vi "ConfigDevice.vi"(8 "error in (no error)":errorcluster, 11 "ChromaAcLoad in":refnum<class "ChromaAcLoad.lvclass">) -> (0 "error out":errorcluster, 3 "ChromaAcLoad out":refnum<class "ChromaAcLoad.lvclass">)   [LabVIEW 2018, in "AcPwrPlugins.lvlib" / "ChromaAcLoad.lvclass"]
doc: "This VI configures the instrument based on the INI file settings or changes to these settings made using the PrefDialog.vi."
uses:
  ChromaAcLoad.lvclass
  TypeDefs/RangeCheck.ctl
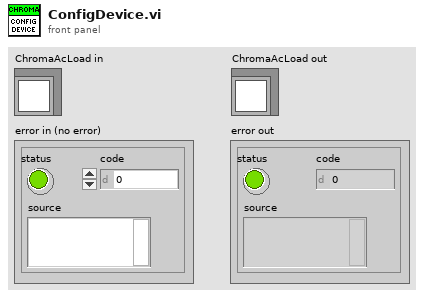
[diagram p1: front panel]
types:
  T1 = enum16{"Constant Voltage (DC)", "Constant Power (DC)", "Constant Power (AC)", "Constant Current (DC)", "Constant Current (AC)", "Constant Resistance (DC)", "Constant Resistance (AC)", "Rectified Mode (DC)", "Inrush (AC)", "RLC CP (AC)", "RLC (AC)"}
  T2 = cluster{"Handle":string, "Name":string, "Phase Select":i32, "Instrument Options":string, "id query (T)":bool, "reset device (T)":bool, "Load Short Circuited":bool, "Line Synchronization":bool, "Load Current (A/Arms)":dbl, "Load Voltage (V/Vrms)":dbl, "Load Power (W)":dbl, "Load Resistance (Ohms)":dbl, "Load Current Peak Limit (A)":dbl, "Load Current Limit (A/Arms)":dbl, "Load Power Limit (W)":dbl, "Synch Frequency (Hz)":dbl, "Priority":enum16{"CF Only", "PF Only", "Both (CF)", "Both (PF)"}, "Crest Factor":dbl, "Power Factor":dbl, "Slew Rate":cluster{"Rise Slew Rate (A/ms)":i32, "Fall Slew Rate (A/ms)":i32}, "LC/RLC Mode":cluster{"Capacitance (uF)":i32, "Inductance (uH)":i32, "Series Resistance (Ohm)":dbl, "Parallel Resistance (Ohm)":dbl}, "Timing":cluster{"TimingOn":enum16{""}, "Hours":u32, "Minutes":u32, "Seconds":dbl, "CutoffVoltage":dbl}, "Connected":bool}[]
  T3 = typedef "AcPwrPlugins.lvlib/ChromaAcLoad.lvclass/RangeCheck.ctl" = enum16{"Power", "Power Limit", "Current", "Current Peak", "Current Limit", "Voltage", "AC Resistance", "DC Resistance", "Frequency", "Crest Factor", "Power Factor", "RLC Power Factor", "Rise Slew Rate", "Fall Slew Rate", "Capacitance", "Inductance", "Parallel Resistance", "Series Resistance"}[]
  T4 = enum16{"CF Only", "PF Only", "Both (CF)", "Both (PF)"}
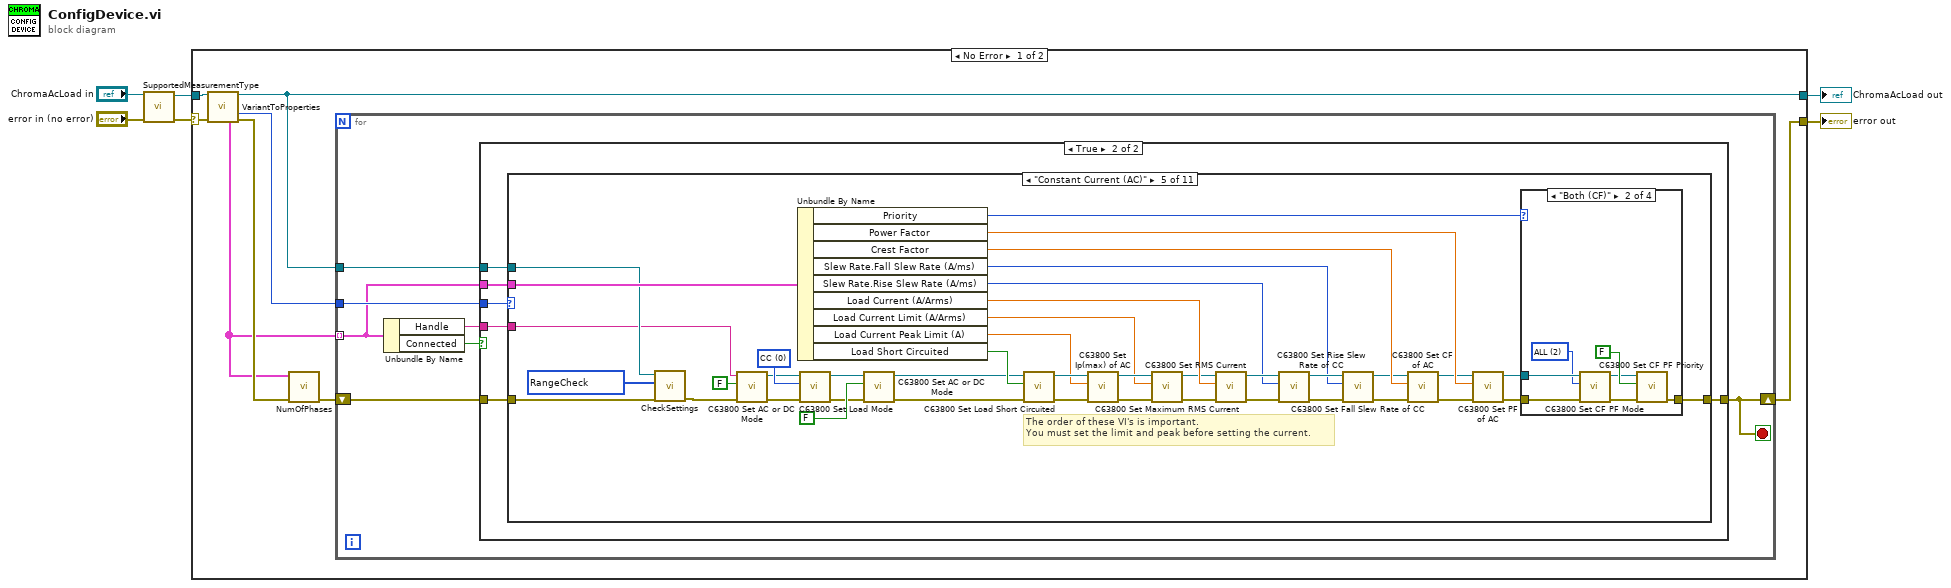
[diagram p0: block diagram]
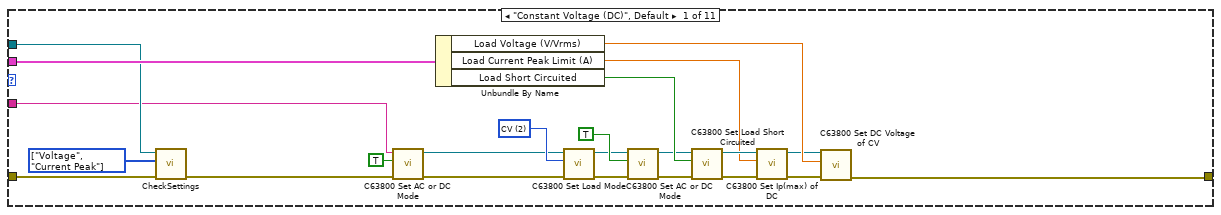
[diagram p3: hidden frame]
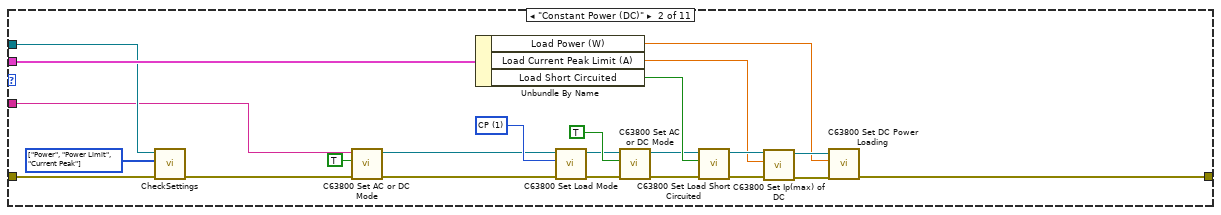
[diagram p4: hidden frame]
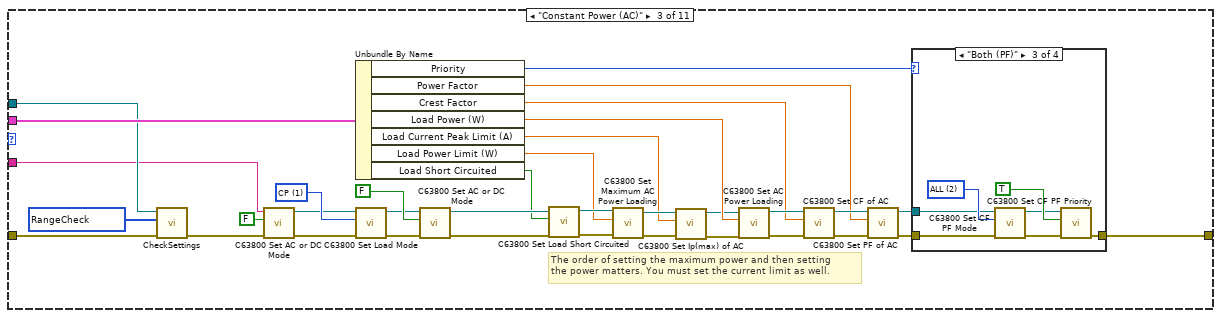
[diagram p5: hidden frame]
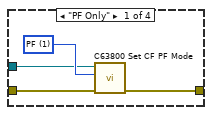
[diagram p6: hidden frame]
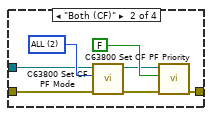
[diagram p7: hidden frame]
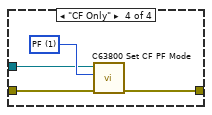
[diagram p8: hidden frame]
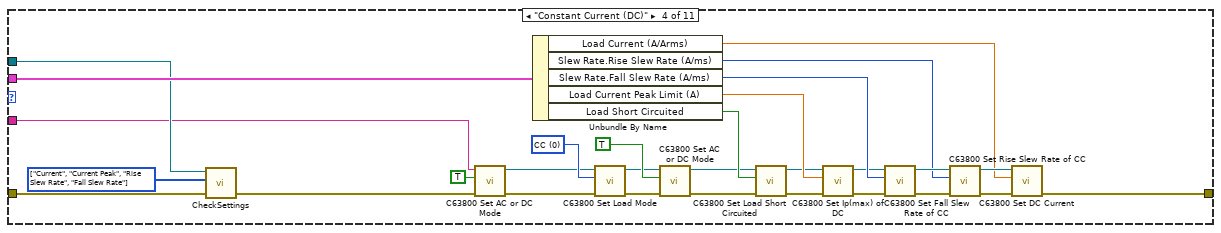
[diagram p9: hidden frame]
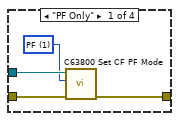
[diagram p10: hidden frame]
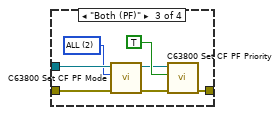
[diagram p11: hidden frame]
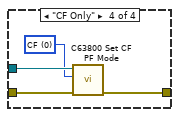
[diagram p12: hidden frame]
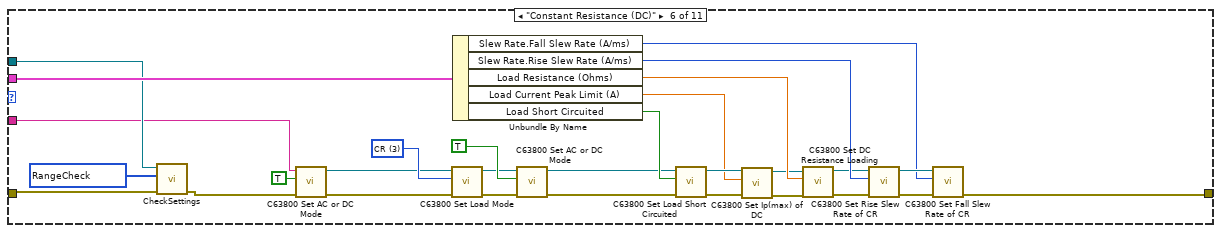
[diagram p13: hidden frame]
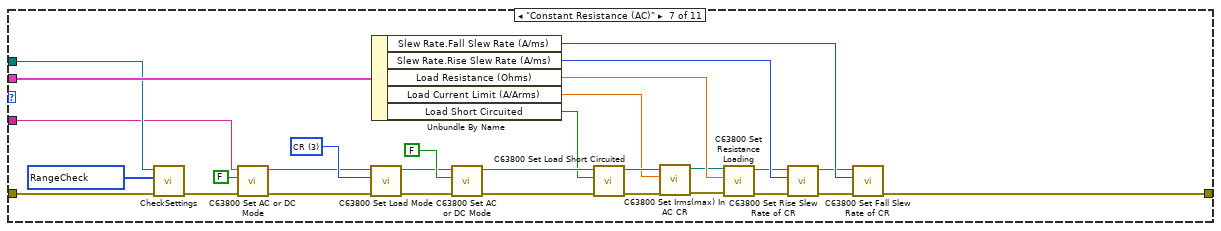
[diagram p14: hidden frame]
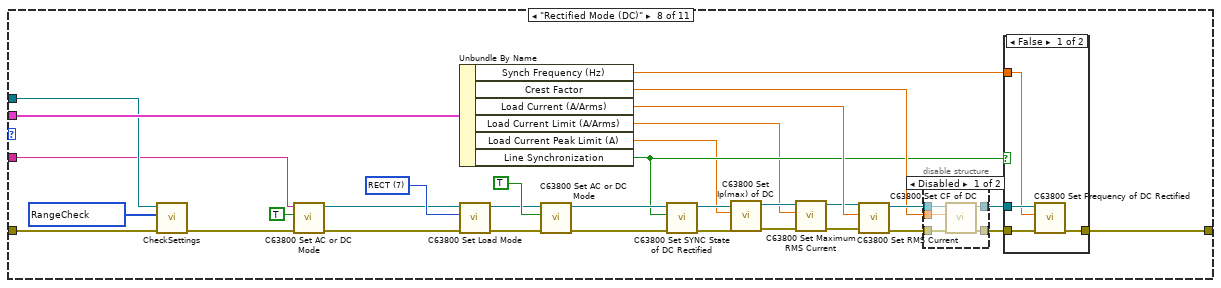
[diagram p15: hidden frame]
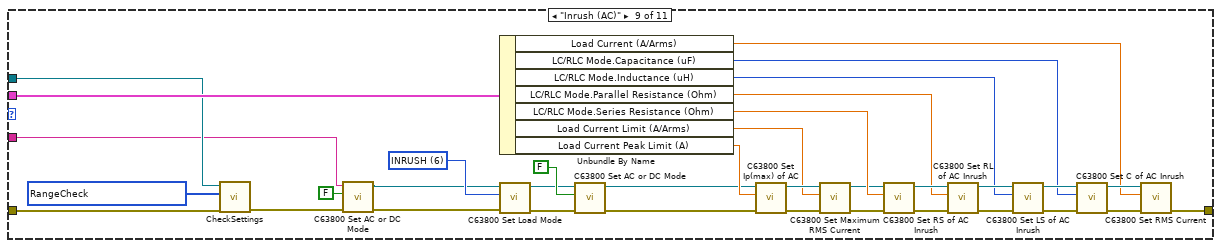
[diagram p18: hidden frame]
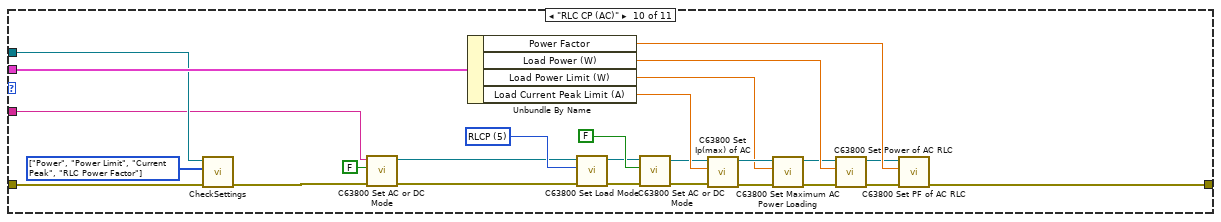
[diagram p19: hidden frame]
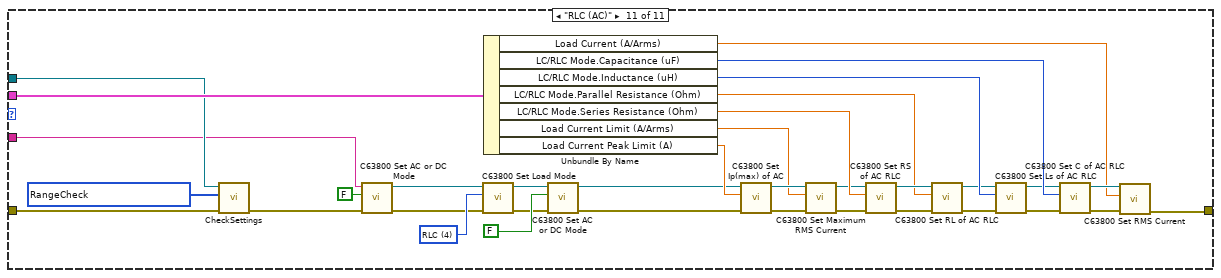
[diagram p20: hidden frame]
diagram:
  n1 = call-dynamic "SupportedMeasurementType.vi"("error in (no error)"="error in (no error)", "ChromaAcLoad in"="ChromaAcLoad in") -> ("error out"=w3:errorcluster, "ChromaAcLoad out"=w4:refnum<class "ChromaAcLoad.lvclass">)  [unwired: 8 in]
  n2 = case shown="No Error" w3 {
    selector: w3 -> [w11 w419]
    tunnel: [w14 w419] -> w6
    tunnel: w4 -> [w13 w418]
    tunnel: [w9 w418] -> w5
    frame No Error {
      n3 = call "VariantToProperties.vi"("ChromaAcLoad"=w13, "error in (no error)"=w11) -> ("ChromaAcLoad"=w9:refnum<class "ChromaAcLoad.lvclass">, "Configuration Mode"=w7:T1, "Phases"=w8:T2, "error out"=w10:errorcluster)  [unwired: 7 in, 3 out]
      n4 = call "NumOfPhases.vi"("Error In"=w10, "Phases"=w8) -> ("Error Out"=w12:errorcluster)  [unwired: 8 in, 1 out]
      n5 = for {
        shift-right: [w18] -> w14
        shift-left: w12 -> [w19]
        tunnel: w8 -> [w16] mode=indexing
        tunnel: w7 -> [w21]
        tunnel: w9 -> [w15]
        stop <- w18 stop-if-true
        n6 = Unbundle By Name(w16) -> ("Handle"=w17:string, "Connected"=w20:bool)
        n7 = case shown="True" w20 {
          tunnel: w21 -> [_ w26]
          tunnel: w19 -> [w22 w28]
          tunnel: [w22 w27] -> w18
          tunnel: w17 -> [_ w25]
          tunnel: w16 -> [_ w24]
          tunnel: w15 -> [_ w23]
          frame False {
          }
          frame True {
            n8 = case shown="\"Constant Current (AC)\"" w26 {
              tunnel: w28 -> [w41 w72 w107 w146 w179 w232 w269 w298 w337 w373 w400]
              tunnel: [w43 w71 w109 w137 w188 w241 w277 w305 w334 w369 w394] -> w27
              tunnel: w25 -> [w31 w54 w75 w130 w159 w221 w250 w278 w325 w357 w383]
              tunnel: w24 -> [w50 w74 w108 w153 w189 w239 w276 w304 w345 w381 w406]
              tunnel: w23 -> [w40 w73 w106 w145 w178 w231 w268 w297 w338 w372 w398]
              frame "Constant Voltage (DC)", Default {
                w39 = T3 [enum."Voltage", enum."Current Peak"] items=["Power", "Power Limit", "Current", "Current Peak", "Current Limit", "Voltage", "AC Resistance", "DC Resistance", "Frequency", "Crest Factor", "Power Factor", "RLC Power Factor", "Rise Slew Rate", "Fall Slew Rate", "Capacitance", "Inductance", "Parallel Resistance", "Series Resistance"] ("RangeCheck")
                w46 = 2 items=["CC", "CP", "CV", "CR", "RLC", "RLCP", "INRUSH", "RECT"] ("Load Mode")
                n9 = call-dynamic "CheckSettings.vi"("ChromaAcLoad in"=w40, "RangeCheck"=w39, "error in (no error)"=w41) -> ("error out"=w33:errorcluster)  [unwired: 6 in, 1 out]
                n10 = call <instrlib>:"C63800 Set AC or DC Mode.vi"("error in (no error)"=w33, "Select AC_DC Mode"=TRUE, "Instrument Handle"=w31) -> ("error out"=w32:errorcluster, "Instrument Handle out"=w30:refnum<k15>)  [unwired: 7 in]
                n11 = Unbundle By Name(w50) -> ("Load Voltage (V/Vrms)"=w42:dbl, "Load Current Peak Limit (A)"=w34:dbl, "Load Short Circuited"=w51:bool)
                n12 = call <instrlib>:"C63800 Set Load Mode.vi"("error in (no error)"=w32, "Load Mode"=w46, "Instrument Handle"=w30) -> ("error out"=w45:errorcluster, "Instrument Handle out"=w44:refnum<k15>)  [unwired: 7 in]
                n13 = call <instrlib>:"C63800 Set AC or DC Mode.vi"("error in (no error)"=w45, "Select AC_DC Mode"=TRUE, "Instrument Handle"=w44) -> ("error out"=w49:errorcluster, "Instrument Handle out"=w47:refnum<k15>)  [unwired: 7 in]
                n14 = call <instrlib>:"C63800 Set Load Short Circuited.vi"("error in (no error)"=w49, "Short Circuited State"=w51, "Instrument Handle"=w47) -> ("error out"=w38:errorcluster, "Instrument Handle out"=w35:refnum<k15>)  [unwired: 7 in]
                n15 = call <instrlib>:"C63800 Set Ip(max) of DC.vi"("error in (no error)"=w38, "I_max_DC"=w34, "Instrument Handle"=w35) -> ("error out"=w36:errorcluster, "Instrument Handle out"=w37:refnum<k15>)  [unwired: 7 in]
                n16 = call <instrlib>:"C63800 Set DC Voltage of CV.vi"("error in (no error)"=w36, "SetDCVoltageofCV"=w42, "Instrument Handle"=w37) -> ("error out"=w43:errorcluster)  [unwired: 7 in, 1 out]
              }
              frame "Constant Power (DC)" {
                w65 = T3 [enum."Power", enum."Power Limit", enum."Current Peak"] items=["Power", "Power Limit", "Current", "Current Peak", "Current Limit", "Voltage", "AC Resistance", "DC Resistance", "Frequency", "Crest Factor", "Power Factor", "RLC Power Factor", "Rise Slew Rate", "Fall Slew Rate", "Capacitance", "Inductance", "Parallel Resistance", "Series Resistance"] ("RangeCheck")
                w68 = 1 items=["CC", "CP", "CV", "CR", "RLC", "RLCP", "INRUSH", "RECT"] ("Load Mode")
                n17 = call-dynamic "CheckSettings.vi"("ChromaAcLoad in"=w73, "RangeCheck"=w65, "error in (no error)"=w72) -> ("error out"=w56:errorcluster)  [unwired: 6 in, 1 out]
                n18 = call <instrlib>:"C63800 Set AC or DC Mode.vi"("error in (no error)"=w56, "Select AC_DC Mode"=TRUE, "Instrument Handle"=w54) -> ("error out"=w55:errorcluster, "Instrument Handle out"=w53:refnum<k15>)  [unwired: 7 in]
                n19 = Unbundle By Name(w74) -> ("Load Power (W)"=w60:dbl, "Load Current Peak Limit (A)"=w59:dbl, "Load Short Circuited"=w70:bool)
                n20 = call <instrlib>:"C63800 Set Load Mode.vi"("error in (no error)"=w55, "Load Mode"=w68, "Instrument Handle"=w53) -> ("error out"=w67:errorcluster, "Instrument Handle out"=w66:refnum<k15>)  [unwired: 7 in]
                n21 = call <instrlib>:"C63800 Set AC or DC Mode.vi"("error in (no error)"=w67, "Select AC_DC Mode"=TRUE, "Instrument Handle"=w66) -> ("error out"=w57:errorcluster, "Instrument Handle out"=w58:refnum<k15>)  [unwired: 7 in]
                n22 = call <instrlib>:"C63800 Set Load Short Circuited.vi"("error in (no error)"=w57, "Short Circuited State"=w70, "Instrument Handle"=w58) -> ("error out"=w64:errorcluster, "Instrument Handle out"=w61:refnum<k15>)  [unwired: 7 in]
                n23 = call <instrlib>:"C63800 Set Ip(max) of DC.vi"("error in (no error)"=w64, "I_max_DC"=w59, "Instrument Handle"=w61) -> ("error out"=w63:errorcluster, "Instrument Handle out"=w62:refnum<k15>)  [unwired: 7 in]
                n24 = call <instrlib>:"C63800 Set DC Power Loading.vi"("error in (no error)"=w63, "DC Power Loading"=w60, "Instrument Handle"=w62) -> ("error out"=w71:errorcluster)  [unwired: 7 in, 1 out]
              }
              frame "Constant Power (AC)" {
                w99 = T3 [enum."Power", enum."Power Limit", enum."Current Peak", enum."Power Factor", enum."Crest Factor"] items=["Power", "Power Limit", "Current", "Current Peak", "Current Limit", "Voltage", "AC Resistance", "DC Resistance", "Frequency", "Crest Factor", "Power Factor", "RLC Power Factor", "Rise Slew Rate", "Fall Slew Rate", "Capacitance", "Inductance", "Parallel Resistance", "Series Resistance"] ("RangeCheck")
                w102 = 1 items=["CC", "CP", "CV", "CR", "RLC", "RLCP", "INRUSH", "RECT"] ("Load Mode")
                # "The order of setting the maximum power and then setting \nthe power matters. You must set the current limit as well."
                n25 = call-dynamic "CheckSettings.vi"("ChromaAcLoad in"=w106, "RangeCheck"=w99, "error in (no error)"=w107) -> ("error out"=w78:errorcluster)  [unwired: 6 in, 1 out]
                n26 = call <instrlib>:"C63800 Set AC or DC Mode.vi"("error in (no error)"=w78, "Select AC_DC Mode"=FALSE, "Instrument Handle"=w75) -> ("error out"=w77:errorcluster, "Instrument Handle out"=w76:refnum<k15>)  [unwired: 7 in]
                n27 = Unbundle By Name(w108) -> ("Priority"=w96:T4, "Power Factor"=w88:dbl, "Crest Factor"=w89:dbl, "Load Power (W)"=w98:dbl, "Load Current Peak Limit (A)"=w83:dbl, "Load Power Limit (W)"=w80:dbl, "Load Short Circuited"=w97:bool)
                n28 = call <instrlib>:"C63800 Set Load Mode.vi"("error in (no error)"=w77, "Load Mode"=w102, "Instrument Handle"=w76) -> ("error out"=w101:errorcluster, "Instrument Handle out"=w100:refnum<k15>)  [unwired: 7 in]
                n29 = call <instrlib>:"C63800 Set AC or DC Mode.vi"("error in (no error)"=w101, "Select AC_DC Mode"=FALSE, "Instrument Handle"=w100) -> ("error out"=w105:errorcluster, "Instrument Handle out"=w104:refnum<k15>)  [unwired: 7 in]
                n30 = call <instrlib>:"C63800 Set Load Short Circuited.vi"("error in (no error)"=w105, "Short Circuited State"=w97, "Instrument Handle"=w104) -> ("error out"=w81:errorcluster, "Instrument Handle out"=w82:refnum<k15>)  [unwired: 7 in]
                n31 = call <instrlib>:"C63800 Set Maximum AC Power Loading.vi"("error in (no error)"=w81, "AC Maximum Power Loading"=w80, "Instrument Handle"=w82) -> ("error out"=w87:errorcluster, "Instrument Handle out"=w84:refnum<k15>)  [unwired: 7 in]
                n32 = call <instrlib>:"C63800 Set Ip(max) of AC.vi"("error in (no error)"=w87, "Current Peak Max"=w83, "Instrument Handle"=w84) -> ("error out"=w86:errorcluster, "Instrument Handle out"=w85:refnum<k15>)  [unwired: 7 in]
                n33 = call <instrlib>:"C63800 Set AC Power Loading.vi"("error in (no error)"=w86, "AC Power Loading"=w98, "Instrument Handle"=w85) -> ("error out"=w93:errorcluster, "Instrument Handle out"=w92:refnum<k15>)  [unwired: 7 in]
                n34 = call <instrlib>:"C63800 Set CF of AC.vi"("error in (no error)"=w93, "CF of AC"=w89, "Instrument Handle"=w92) -> ("error out"=w95:errorcluster, "Instrument Handle out"=w94:refnum<k15>)  [unwired: 7 in]
                n35 = call <instrlib>:"C63800 Set PF of AC.vi"("error in (no error)"=w95, "PF of AC"=w88, "Instrument Handle"=w94) -> ("error out"=w91:errorcluster, "Instrument Handle out"=w90:refnum<k15>)  [unwired: 7 in]
                n36 = case shown="\"Both (PF)\"" w96 {
                  tunnel: [w112 w117 w123 w128] -> w109
                  tunnel: w91 -> [w111 w115 w120 w126]
                  tunnel: w90 -> [w110 w114 w121 w127]
                  frame "PF Only" {
                    w113 = 1 items=["CF", "PF", "ALL"] ("CF_PF Mode")
                    n37 = call <instrlib>:"C63800 Set CF PF Mode.vi"("error in (no error)"=w111, "CF_PF Mode"=w113, "Instrument Handle"=w110) -> ("error out"=w112:errorcluster)  [unwired: 7 in, 1 out]
                  }
                  frame "Both (CF)" {
                    w119 = 2 items=["CF", "PF", "ALL"] ("CF_PF Mode")
                    n38 = call <instrlib>:"C63800 Set CF PF Mode.vi"("error in (no error)"=w115, "CF_PF Mode"=w119, "Instrument Handle"=w114) -> ("error out"=w117:errorcluster, "Instrument Handle out"=w116:refnum<k15>)  [unwired: 7 in]
                    n39 = call <instrlib>:"C63800 Set CF PF Priority.vi"("error in (no error)"=w117, "Priority"=FALSE, "Instrument Handle"=w116) -> ()  [unwired: 7 in, 2 out]
                  }
                  frame "Both (PF)" {
                    w125 = 2 items=["CF", "PF", "ALL"] ("CF_PF Mode")
                    n40 = call <instrlib>:"C63800 Set CF PF Mode.vi"("error in (no error)"=w120, "CF_PF Mode"=w125, "Instrument Handle"=w121) -> ("error out"=w123:errorcluster, "Instrument Handle out"=w122:refnum<k15>)  [unwired: 7 in]
                    n41 = call <instrlib>:"C63800 Set CF PF Priority.vi"("error in (no error)"=w123, "Priority"=TRUE, "Instrument Handle"=w122) -> ()  [unwired: 7 in, 2 out]
                  }
                  frame "CF Only" {
                    w129 = 1 items=["CF", "PF", "ALL"] ("CF_PF Mode")
                    n42 = call <instrlib>:"C63800 Set CF PF Mode.vi"("error in (no error)"=w126, "CF_PF Mode"=w129, "Instrument Handle"=w127) -> ("error out"=w128:errorcluster)  [unwired: 7 in, 1 out]
                  }
                }
              }
              frame "Constant Current (DC)" {
                w135 = T3 [enum."Current", enum."Current Peak", enum."Rise Slew Rate", enum."Fall Slew Rate"] items=["Power", "Power Limit", "Current", "Current Peak", "Current Limit", "Voltage", "AC Resistance", "DC Resistance", "Frequency", "Crest Factor", "Power Factor", "RLC Power Factor", "Rise Slew Rate", "Fall Slew Rate", "Capacitance", "Inductance", "Parallel Resistance", "Series Resistance"] ("RangeCheck")
                w150 = 0 items=["CC", "CP", "CV", "CR", "RLC", "RLCP", "INRUSH", "RECT"] ("Load Mode")
                n43 = call-dynamic "CheckSettings.vi"("ChromaAcLoad in"=w145, "RangeCheck"=w135, "error in (no error)"=w146) -> ("error out"=w131:errorcluster)  [unwired: 6 in, 1 out]
                n44 = call <instrlib>:"C63800 Set AC or DC Mode.vi"("error in (no error)"=w131, "Select AC_DC Mode"=TRUE, "Instrument Handle"=w130) -> ("error out"=w133:errorcluster, "Instrument Handle out"=w132:refnum<k15>)  [unwired: 7 in]
                n45 = Unbundle By Name(w153) -> ("Load Current (A/Arms)"=w136:dbl, "Slew Rate.Rise Slew Rate (A/ms)"=w155:i32, "Slew Rate.Fall Slew Rate (A/ms)"=w156:i32, "Load Current Peak Limit (A)"=w141:dbl, "Load Short Circuited"=w154:bool)
                n46 = call <instrlib>:"C63800 Set Load Mode.vi"("error in (no error)"=w133, "Load Mode"=w150, "Instrument Handle"=w132) -> ("error out"=w149:errorcluster, "Instrument Handle out"=w148:refnum<k15>)  [unwired: 7 in]
                n47 = call <instrlib>:"C63800 Set AC or DC Mode.vi"("error in (no error)"=w149, "Select AC_DC Mode"=TRUE, "Instrument Handle"=w148) -> ("error out"=w147:errorcluster, "Instrument Handle out"=w151:refnum<k15>)  [unwired: 7 in]
                n48 = call <instrlib>:"C63800 Set Load Short Circuited.vi"("error in (no error)"=w147, "Short Circuited State"=w154, "Instrument Handle"=w151) -> ("error out"=w144:errorcluster, "Instrument Handle out"=w140:refnum<k15>)  [unwired: 7 in]
                n49 = call <instrlib>:"C63800 Set Ip(max) of DC.vi"("error in (no error)"=w144, "I_max_DC"=w141, "Instrument Handle"=w140) -> ("error out"=w143:errorcluster, "Instrument Handle out"=w142:refnum<k15>)  [unwired: 7 in]
                n50 = call <instrlib>:"C63800 Set Fall Slew Rate of CC.vi"("error in (no error)"=w143, "Fall Slew Rate of CC"=w156, "Instrument Handle"=w142) -> ("error out"=w158:errorcluster, "Instrument Handle out"=w157:refnum<k15>)  [unwired: 7 in]
                n51 = call <instrlib>:"C63800 Set Rise Slew Rate of CC.vi"("error in (no error)"=w158, "Rise Slew Rate of CC"=w155, "Instrument Handle"=w157) -> ("error out"=w139:errorcluster, "Instrument Handle out"=w138:refnum<k15>)  [unwired: 7 in]
                n52 = call <instrlib>:"C63800 Set DC Current.vi"("error in (no error)"=w139, "Set DC Current"=w136, "Instrument Handle"=w138) -> ("error out"=w137:errorcluster)  [unwired: 7 in, 1 out]
              }
              frame "Constant Current (AC)" {
                w177 = T3 [enum."Current", enum."Current Peak", enum."Current Limit", enum."Power Factor", enum."Crest Factor", enum."Fall Slew Rate", enum."Rise Slew Rate"] items=["Power", "Power Limit", "Current", "Current Peak", "Current Limit", "Voltage", "AC Resistance", "DC Resistance", "Frequency", "Crest Factor", "Power Factor", "RLC Power Factor", "Rise Slew Rate", "Fall Slew Rate", "Capacitance", "Inductance", "Parallel Resistance", "Series Resistance"] ("RangeCheck")
                w185 = 0 items=["CC", "CP", "CV", "CR", "RLC", "RLCP", "INRUSH", "RECT"] ("Load Mode")
                # "The order of these VI's is important. \nYou must set the limit and peak before setting the current."
                n53 = call-dynamic "CheckSettings.vi"("ChromaAcLoad in"=w178, "RangeCheck"=w177, "error in (no error)"=w179) -> ("error out"=w162:errorcluster)  [unwired: 6 in, 1 out]
                n54 = call <instrlib>:"C63800 Set AC or DC Mode.vi"("error in (no error)"=w162, "Select AC_DC Mode"=FALSE, "Instrument Handle"=w159) -> ("error out"=w161:errorcluster, "Instrument Handle out"=w160:refnum<k15>)  [unwired: 7 in]
                n55 = Unbundle By Name(w189) -> ("Priority"=w195:T4, "Power Factor"=w198:dbl, "Crest Factor"=w197:dbl, "Slew Rate.Fall Slew Rate (A/ms)"=w169:i32, "Slew Rate.Rise Slew Rate (A/ms)"=w170:i32, "Load Current (A/Arms)"=w181:dbl, "Load Current Limit (A/Arms)"=w164:dbl, "Load Current Peak Limit (A)"=w165:dbl, "Load Short Circuited"=w190:bool)
                n56 = call <instrlib>:"C63800 Set Load Mode.vi"("error in (no error)"=w161, "Load Mode"=w185, "Instrument Handle"=w160) -> ("error out"=w184:errorcluster, "Instrument Handle out"=w183:refnum<k15>)  [unwired: 7 in]
                n57 = call <instrlib>:"C63800 Set AC or DC Mode.vi"("error in (no error)"=w184, "Select AC_DC Mode"=FALSE, "Instrument Handle"=w183) -> ("error out"=w180:errorcluster, "Instrument Handle out"=w186:refnum<k15>)  [unwired: 7 in]
                n58 = call <instrlib>:"C63800 Set Load Short Circuited.vi"("error in (no error)"=w180, "Short Circuited State"=w190, "Instrument Handle"=w186) -> ("error out"=w191:errorcluster, "Instrument Handle out"=w192:refnum<k15>)  [unwired: 7 in]
                n59 = call <instrlib>:"C63800 Set Ip(max) of AC.vi"("error in (no error)"=w191, "Current Peak Max"=w165, "Instrument Handle"=w192) -> ("error out"=w182:errorcluster, "Instrument Handle out"=w167:refnum<k15>)  [unwired: 7 in]
                n60 = call <instrlib>:"C63800 Set Maximum RMS Current.vi"("error in (no error)"=w182, "Set Max RMS Current"=w164, "Instrument Handle"=w167) -> ("error out"=w168:errorcluster, "Instrument Handle out"=w166:refnum<k15>)  [unwired: 7 in]
                n61 = call <instrlib>:"C63800 Set RMS Current.vi"("error in (no error)"=w168, "Set RMS Current"=w181, "Instrument Handle"=w166) -> ("error out"=w176:errorcluster, "Instrument Handle out"=w175:refnum<k15>)  [unwired: 7 in]
                n62 = call <instrlib>:"C63800 Set Rise Slew Rate of CC.vi"("error in (no error)"=w176, "Rise Slew Rate of CC"=w170, "Instrument Handle"=w175) -> ("error out"=w174:errorcluster, "Instrument Handle out"=w173:refnum<k15>)  [unwired: 7 in]
                n63 = call <instrlib>:"C63800 Set Fall Slew Rate of CC.vi"("error in (no error)"=w174, "Fall Slew Rate of CC"=w169, "Instrument Handle"=w173) -> ("error out"=w171:errorcluster, "Instrument Handle out"=w172:refnum<k15>)  [unwired: 7 in]
                n64 = call <instrlib>:"C63800 Set CF of AC.vi"("error in (no error)"=w171, "CF of AC"=w197, "Instrument Handle"=w172) -> ("error out"=w199:errorcluster, "Instrument Handle out"=w196:refnum<k15>)  [unwired: 7 in]
                n65 = call <instrlib>:"C63800 Set PF of AC.vi"("error in (no error)"=w199, "PF of AC"=w198, "Instrument Handle"=w196) -> ("error out"=w193:errorcluster, "Instrument Handle out"=w194:refnum<k15>)  [unwired: 7 in]
                n66 = case shown="\"Both (CF)\"" w195 {
                  tunnel: w194 -> [w203 w209 w215 w219]
                  tunnel: w193 -> [w202 w208 w214 w218]
                  tunnel: [w200 w205 w211 w216] -> w188
                  frame "PF Only" {
                    w201 = 1 items=["CF", "PF", "ALL"] ("CF_PF Mode")
                    n67 = call <instrlib>:"C63800 Set CF PF Mode.vi"("error in (no error)"=w202, "CF_PF Mode"=w201, "Instrument Handle"=w203) -> ("error out"=w200:errorcluster)  [unwired: 7 in, 1 out]
                  }
                  frame "Both (CF)" {
                    w207 = 2 items=["CF", "PF", "ALL"] ("CF_PF Mode")
                    n68 = call <instrlib>:"C63800 Set CF PF Mode.vi"("error in (no error)"=w208, "CF_PF Mode"=w207, "Instrument Handle"=w209) -> ("error out"=w205:errorcluster, "Instrument Handle out"=w204:refnum<k15>)  [unwired: 7 in]
                    n69 = call <instrlib>:"C63800 Set CF PF Priority.vi"("error in (no error)"=w205, "Priority"=FALSE, "Instrument Handle"=w204) -> ()  [unwired: 7 in, 2 out]
                  }
                  frame "Both (PF)" {
                    w213 = 2 items=["CF", "PF", "ALL"] ("CF_PF Mode")
                    n70 = call <instrlib>:"C63800 Set CF PF Mode.vi"("error in (no error)"=w214, "CF_PF Mode"=w213, "Instrument Handle"=w215) -> ("error out"=w211:errorcluster, "Instrument Handle out"=w210:refnum<k15>)  [unwired: 7 in]
                    n71 = call <instrlib>:"C63800 Set CF PF Priority.vi"("error in (no error)"=w211, "Priority"=TRUE, "Instrument Handle"=w210) -> ()  [unwired: 7 in, 2 out]
                  }
                  frame "CF Only" {
                    w217 = 0 items=["CF", "PF", "ALL"] ("CF_PF Mode")
                    n72 = call <instrlib>:"C63800 Set CF PF Mode.vi"("error in (no error)"=w218, "CF_PF Mode"=w217, "Instrument Handle"=w219) -> ("error out"=w216:errorcluster)  [unwired: 7 in, 1 out]
                  }
                }
              }
              frame "Constant Resistance (DC)" {
                w230 = T3 [enum."DC Resistance", enum."Current Peak", enum."Rise Slew Rate", enum."Fall Slew Rate"] items=["Power", "Power Limit", "Current", "Current Peak", "Current Limit", "Voltage", "AC Resistance", "DC Resistance", "Frequency", "Crest Factor", "Power Factor", "RLC Power Factor", "Rise Slew Rate", "Fall Slew Rate", "Capacitance", "Inductance", "Parallel Resistance", "Series Resistance"] ("RangeCheck")
                w236 = 3 items=["CC", "CP", "CV", "CR", "RLC", "RLCP", "INRUSH", "RECT"] ("Load Mode")
                n73 = call-dynamic "CheckSettings.vi"("ChromaAcLoad in"=w231, "RangeCheck"=w230, "error in (no error)"=w232) -> ("error out"=w223:errorcluster)  [unwired: 6 in, 1 out]
                n74 = call <instrlib>:"C63800 Set AC or DC Mode.vi"("error in (no error)"=w223, "Select AC_DC Mode"=TRUE, "Instrument Handle"=w221) -> ("error out"=w222:errorcluster, "Instrument Handle out"=w220:refnum<k15>)  [unwired: 7 in]
                n75 = call <instrlib>:"C63800 Set Load Mode.vi"("error in (no error)"=w222, "Load Mode"=w236, "Instrument Handle"=w220) -> ("error out"=w235:errorcluster, "Instrument Handle out"=w234:refnum<k15>)  [unwired: 7 in]
                n76 = Unbundle By Name(w239) -> ("Slew Rate.Fall Slew Rate (A/ms)"=w245:i32, "Slew Rate.Rise Slew Rate (A/ms)"=w244:i32, "Load Resistance (Ohms)"=w248:dbl, "Load Current Peak Limit (A)"=w225:dbl, "Load Short Circuited"=w240:bool)
                n77 = call <instrlib>:"C63800 Set AC or DC Mode.vi"("error in (no error)"=w235, "Select AC_DC Mode"=TRUE, "Instrument Handle"=w234) -> ("error out"=w233:errorcluster, "Instrument Handle out"=w238:refnum<k15>)  [unwired: 7 in]
                n78 = call <instrlib>:"C63800 Set Load Short Circuited.vi"("error in (no error)"=w233, "Short Circuited State"=w240, "Instrument Handle"=w238) -> ("error out"=w227:errorcluster, "Instrument Handle out"=w226:refnum<k15>)  [unwired: 7 in]
                n79 = call <instrlib>:"C63800 Set Ip(max) of DC.vi"("error in (no error)"=w227, "I_max_DC"=w225, "Instrument Handle"=w226) -> ("error out"=w229:errorcluster, "Instrument Handle out"=w228:refnum<k15>)  [unwired: 7 in]
                n80 = call <instrlib>:"C63800 Set DC Resistance Loading.vi"("error in (no error)"=w229, "DC Resistance Loading"=w248, "Instrument Handle"=w228) -> ("error out"=w242:errorcluster, "Instrument Handle out"=w243:refnum<k15>)  [unwired: 7 in]
                n81 = call <instrlib>:"C63800 Set Rise Slew Rate of CR.vi"("error in (no error)"=w242, "Rise Slew Rate of CR"=w244, "Instrument Handle"=w243) -> ("error out"=w246:errorcluster, "Instrument Handle out"=w247:refnum<k15>)  [unwired: 7 in]
                n82 = call <instrlib>:"C63800 Set Fall Slew Rate of CR.vi"("error in (no error)"=w246, "Fall Slew Rate of CR"=w245, "Instrument Handle"=w247) -> ("error out"=w241:errorcluster)  [unwired: 7 in, 1 out]
              }
              frame "Constant Resistance (AC)" {
                w267 = T3 [enum."AC Resistance", enum."Current Limit", enum."Rise Slew Rate", enum."Fall Slew Rate"] items=["Power", "Power Limit", "Current", "Current Peak", "Current Limit", "Voltage", "AC Resistance", "DC Resistance", "Frequency", "Crest Factor", "Power Factor", "RLC Power Factor", "Rise Slew Rate", "Fall Slew Rate", "Capacitance", "Inductance", "Parallel Resistance", "Series Resistance"] ("RangeCheck")
                w273 = 3 items=["CC", "CP", "CV", "CR", "RLC", "RLCP", "INRUSH", "RECT"] ("Load Mode")
                n83 = call-dynamic "CheckSettings.vi"("ChromaAcLoad in"=w268, "RangeCheck"=w267, "error in (no error)"=w269) -> ("error out"=w252:errorcluster)  [unwired: 6 in, 1 out]
                n84 = call <instrlib>:"C63800 Set AC or DC Mode.vi"("error in (no error)"=w252, "Select AC_DC Mode"=FALSE, "Instrument Handle"=w250) -> ("error out"=w251:errorcluster, "Instrument Handle out"=w249:refnum<k15>)  [unwired: 7 in]
                n85 = call <instrlib>:"C63800 Set Load Mode.vi"("error in (no error)"=w251, "Load Mode"=w273, "Instrument Handle"=w249) -> ("error out"=w272:errorcluster, "Instrument Handle out"=w271:refnum<k15>)  [unwired: 7 in]
                n86 = Unbundle By Name(w276) -> ("Slew Rate.Fall Slew Rate (A/ms)"=w260:i32, "Slew Rate.Rise Slew Rate (A/ms)"=w262:i32, "Load Resistance (Ohms)"=w263:dbl, "Load Current Limit (A/Arms)"=w254:dbl, "Load Short Circuited"=w264:bool)
                n87 = call <instrlib>:"C63800 Set AC or DC Mode.vi"("error in (no error)"=w272, "Select AC_DC Mode"=FALSE, "Instrument Handle"=w271) -> ("error out"=w270:errorcluster, "Instrument Handle out"=w275:refnum<k15>)  [unwired: 7 in]
                n88 = call <instrlib>:"C63800 Set Load Short Circuited.vi"("error in (no error)"=w270, "Short Circuited State"=w264, "Instrument Handle"=w275) -> ("error out"=w258:errorcluster, "Instrument Handle out"=w257:refnum<k15>)  [unwired: 7 in]
                n89 = call <instrlib>:"C63800 Set Irms(max) In AC CR.vi"("error in (no error)"=w258, "I_max"=w254, "Instrument Handle"=w257) -> ("error out"=w255:errorcluster, "Instrument Handle out"=w256:refnum<k15>)  [unwired: 7 in]
                n90 = call <instrlib>:"C63800 Set Resistance Loading.vi"("error in (no error)"=w255, "Resistance Loading"=w263, "Instrument Handle"=w256) -> ("error out"=w265:errorcluster, "Instrument Handle out"=w261:refnum<k15>)  [unwired: 7 in]
                n91 = call <instrlib>:"C63800 Set Rise Slew Rate of CR.vi"("error in (no error)"=w265, "Rise Slew Rate of CR"=w262, "Instrument Handle"=w261) -> ("error out"=w266:errorcluster, "Instrument Handle out"=w259:refnum<k15>)  [unwired: 7 in]
                n92 = call <instrlib>:"C63800 Set Fall Slew Rate of CR.vi"("error in (no error)"=w266, "Fall Slew Rate of CR"=w260, "Instrument Handle"=w259) -> ("error out"=w277:errorcluster)  [unwired: 7 in, 1 out]
              }
              frame "Rectified Mode (DC)" {
                w296 = T3 [enum."Current", enum."Current Peak", enum."Current Limit", enum."Crest Factor", enum."Frequency"] items=["Power", "Power Limit", "Current", "Current Peak", "Current Limit", "Voltage", "AC Resistance", "DC Resistance", "Frequency", "Crest Factor", "Power Factor", "RLC Power Factor", "Rise Slew Rate", "Fall Slew Rate", "Capacitance", "Inductance", "Parallel Resistance", "Series Resistance"] ("RangeCheck")
                w301 = 7 items=["CC", "CP", "CV", "CR", "RLC", "RLCP", "INRUSH", "RECT"] ("Load Mode")
                n93 = call-dynamic "CheckSettings.vi"("ChromaAcLoad in"=w297, "RangeCheck"=w296, "error in (no error)"=w298) -> ("error out"=w281:errorcluster)  [unwired: 6 in, 1 out]
                n94 = call <instrlib>:"C63800 Set AC or DC Mode.vi"("error in (no error)"=w281, "Select AC_DC Mode"=TRUE, "Instrument Handle"=w278) -> ("error out"=w280:errorcluster, "Instrument Handle out"=w279:refnum<k15>)  [unwired: 7 in]
                n95 = Unbundle By Name(w304) -> ("Synch Frequency (Hz)"=w285:dbl, "Crest Factor"=w295:dbl, "Load Current (A/Arms)"=w303:dbl, "Load Current Limit (A/Arms)"=w283:dbl, "Load Current Peak Limit (A)"=w284:dbl, "Line Synchronization"=w286:bool)
                n96 = call <instrlib>:"C63800 Set Load Mode.vi"("error in (no error)"=w280, "Load Mode"=w301, "Instrument Handle"=w279) -> ("error out"=w300:errorcluster, "Instrument Handle out"=w299:refnum<k15>)  [unwired: 7 in]
                n97 = call <instrlib>:"C63800 Set AC or DC Mode.vi"("error in (no error)"=w300, "Select AC_DC Mode"=TRUE, "Instrument Handle"=w299) -> ("error out"=w294:errorcluster, "Instrument Handle out"=w292:refnum<k15>)  [unwired: 7 in]
                n98 = call <instrlib>:"C63800 Set SYNC State of DC Rectified.vi"("error in (no error)"=w294, "SYNC State of DC Rectified"=w286, "Instrument Handle"=w292) -> ("error out"=w293:errorcluster, "Instrument Handle out"=w291:refnum<k15>)  [unwired: 7 in]
                n99 = call <instrlib>:"C63800 Set Ip(max) of DC.vi"("error in (no error)"=w293, "I_max_DC"=w284, "Instrument Handle"=w291) -> ("error out"=w288:errorcluster, "Instrument Handle out"=w287:refnum<k15>)  [unwired: 7 in]
                n100 = call <instrlib>:"C63800 Set Maximum RMS Current.vi"("error in (no error)"=w288, "Set Max RMS Current"=w283, "Instrument Handle"=w287) -> ("error out"=w290:errorcluster, "Instrument Handle out"=w289:refnum<k15>)  [unwired: 7 in]
                n101 = call <instrlib>:"C63800 Set RMS Current.vi"("error in (no error)"=w290, "Set RMS Current"=w303, "Instrument Handle"=w289) -> ("error out"=w309:errorcluster, "Instrument Handle out"=w308:refnum<k15>)  [unwired: 7 in]
                n102 = disable-structure shown="Disabled" {
                  disable-tunnel: w309 -> [w314 w315]
                  disable-tunnel: w308 -> [w313 w316]
                  disable-tunnel: [w312 w316] -> w307
                  disable-tunnel: [w311 w315] -> w306
                  disable-tunnel: w295 -> [w310 _]
                  frame Disabled {
                    n103 = call <instrlib>:"C63800 Set CF of DC.vi"("error in (no error)"=w314, "CF of DC"=w310, "Instrument Handle"=w313) -> ("error out"=w311:errorcluster, "Instrument Handle out"=w312:refnum<k15>)  [unwired: 7 in]
                  }
                  frame Enabled {
                  }
                }
                n104 = case shown="False" w286 {
                  tunnel: w307 -> [w320 _]
                  tunnel: w306 -> [w319 w321]
                  tunnel: [w318 w321] -> w305
                  tunnel: w285 -> [w317 _]
                  frame False {
                    n105 = call <instrlib>:"C63800 Set Frequency of DC Rectified.vi"("error in (no error)"=w319, "Frequency of DC Rectified"=w317, "Instrument Handle"=w320) -> ("error out"=w318:errorcluster)  [unwired: 7 in, 1 out]
                  }
                  frame True {
                  }
                }
              }
              frame "Inrush (AC)" {
                w336 = T3 [enum."Current", enum."Current Peak", enum."Current Limit", enum."Capacitance", enum."Inductance", enum."Current", enum."Parallel Resistance", enum."Series Resistance"] items=["Power", "Power Limit", "Current", "Current Peak", "Current Limit", "Voltage", "AC Resistance", "DC Resistance", "Frequency", "Crest Factor", "Power Factor", "RLC Power Factor", "Rise Slew Rate", "Fall Slew Rate", "Capacitance", "Inductance", "Parallel Resistance", "Series Resistance"] ("RangeCheck")
                w341 = 6 items=["CC", "CP", "CV", "CR", "RLC", "RLCP", "INRUSH", "RECT"] ("Load Mode")
                n106 = call-dynamic "CheckSettings.vi"("ChromaAcLoad in"=w338, "RangeCheck"=w336, "error in (no error)"=w337) -> ("error out"=w324:errorcluster)  [unwired: 6 in, 1 out]
                n107 = call <instrlib>:"C63800 Set AC or DC Mode.vi"("error in (no error)"=w324, "Select AC_DC Mode"=FALSE, "Instrument Handle"=w325) -> ("error out"=w322:errorcluster, "Instrument Handle out"=w323:refnum<k15>)  [unwired: 7 in]
                n108 = Unbundle By Name(w345) -> ("Load Current (A/Arms)"=w332:dbl, "LC/RLC Mode.Capacitance (uF)"=w350:i32, "LC/RLC Mode.Inductance (uH)"=w349:i32, "LC/RLC Mode.Parallel Resistance (Ohm)"=w348:dbl, "LC/RLC Mode.Series Resistance (Ohm)"=w347:dbl, "Load Current Limit (A/Arms)"=w327:dbl, "Load Current Peak Limit (A)"=w346:dbl)
                n109 = call <instrlib>:"C63800 Set Load Mode.vi"("error in (no error)"=w322, "Load Mode"=w341, "Instrument Handle"=w323) -> ("error out"=w340:errorcluster, "Instrument Handle out"=w339:refnum<k15>)  [unwired: 7 in]
                n110 = call <instrlib>:"C63800 Set AC or DC Mode.vi"("error in (no error)"=w340, "Select AC_DC Mode"=FALSE, "Instrument Handle"=w339) -> ("error out"=w344:errorcluster, "Instrument Handle out"=w343:refnum<k15>)  [unwired: 7 in]
                n111 = call <instrlib>:"C63800 Set Ip(max) of AC.vi"("error in (no error)"=w344, "Current Peak Max"=w346, "Instrument Handle"=w343) -> ("error out"=w329:errorcluster, "Instrument Handle out"=w328:refnum<k15>)  [unwired: 7 in]
                n112 = call <instrlib>:"C63800 Set Maximum RMS Current.vi"("error in (no error)"=w329, "Set Max RMS Current"=w327, "Instrument Handle"=w328) -> ("error out"=w331:errorcluster, "Instrument Handle out"=w330:refnum<k15>)  [unwired: 7 in]
                n113 = call <instrlib>:"C63800 Set RS of AC Inrush.vi"("error in (no error)"=w331, "RS of AC Inrush"=w347, "Instrument Handle"=w330) -> ("error out"=w352:errorcluster, "Instrument Handle out"=w351:refnum<k15>)  [unwired: 7 in]
                n114 = call <instrlib>:"C63800 Set RL of AC Inrush.vi"("error in (no error)"=w352, "RL of AC Inrush"=w348, "Instrument Handle"=w351) -> ("error out"=w356:errorcluster, "Instrument Handle out"=w355:refnum<k15>)  [unwired: 7 in]
                n115 = call <instrlib>:"C63800 Set LS of AC Inrush.vi"("error in (no error)"=w356, "LS of AC Inrush"=w349, "Instrument Handle"=w355) -> ("error out"=w354:errorcluster, "Instrument Handle out"=w353:refnum<k15>)  [unwired: 7 in]
                n116 = call <instrlib>:"C63800 Set C of AC Inrush.vi"("error in (no error)"=w354, "C of AC Inrush"=w350, "Instrument Handle"=w353) -> ("error out"=w335:errorcluster, "Instrument Handle out"=w333:refnum<k15>)  [unwired: 7 in]
                n117 = call <instrlib>:"C63800 Set RMS Current.vi"("error in (no error)"=w335, "Set RMS Current"=w332, "Instrument Handle"=w333) -> ("error out"=w334:errorcluster)  [unwired: 7 in, 1 out]
              }
              frame "RLC CP (AC)" {
                w371 = T3 [enum."Power", enum."Power Limit", enum."Current Peak", enum."RLC Power Factor"] items=["Power", "Power Limit", "Current", "Current Peak", "Current Limit", "Voltage", "AC Resistance", "DC Resistance", "Frequency", "Crest Factor", "Power Factor", "RLC Power Factor", "Rise Slew Rate", "Fall Slew Rate", "Capacitance", "Inductance", "Parallel Resistance", "Series Resistance"] ("RangeCheck")
                w376 = 5 items=["CC", "CP", "CV", "CR", "RLC", "RLCP", "INRUSH", "RECT"] ("Load Mode")
                n118 = call-dynamic "CheckSettings.vi"("ChromaAcLoad in"=w372, "RangeCheck"=w371, "error in (no error)"=w373) -> ("error out"=w360:errorcluster)  [unwired: 6 in, 1 out]
                n119 = call <instrlib>:"C63800 Set AC or DC Mode.vi"("error in (no error)"=w360, "Select AC_DC Mode"=FALSE, "Instrument Handle"=w357) -> ("error out"=w359:errorcluster, "Instrument Handle out"=w358:refnum<k15>)  [unwired: 7 in]
                n120 = Unbundle By Name(w381) -> ("Power Factor"=w368:dbl, "Load Power (W)"=w382:dbl, "Load Power Limit (W)"=w362:dbl, "Load Current Peak Limit (A)"=w380:dbl)
                n121 = call <instrlib>:"C63800 Set Load Mode.vi"("error in (no error)"=w359, "Load Mode"=w376, "Instrument Handle"=w358) -> ("error out"=w375:errorcluster, "Instrument Handle out"=w374:refnum<k15>)  [unwired: 7 in]
                n122 = call <instrlib>:"C63800 Set AC or DC Mode.vi"("error in (no error)"=w375, "Select AC_DC Mode"=FALSE, "Instrument Handle"=w374) -> ("error out"=w379:errorcluster, "Instrument Handle out"=w378:refnum<k15>)  [unwired: 7 in]
                n123 = call <instrlib>:"C63800 Set Ip(max) of AC.vi"("error in (no error)"=w379, "Current Peak Max"=w380, "Instrument Handle"=w378) -> ("error out"=w363:errorcluster, "Instrument Handle out"=w364:refnum<k15>)  [unwired: 7 in]
                n124 = call <instrlib>:"C63800 Set Maximum AC Power Loading.vi"("error in (no error)"=w363, "AC Maximum Power Loading"=w362, "Instrument Handle"=w364) -> ("error out"=w366:errorcluster, "Instrument Handle out"=w365:refnum<k15>)  [unwired: 7 in]
                n125 = call <instrlib>:"C63800 Set Power of AC RLC.vi"("error in (no error)"=w366, "Power of RLC"=w382, "Instrument Handle"=w365) -> ("error out"=w370:errorcluster, "Instrument Handle out"=w367:refnum<k15>)  [unwired: 7 in]
                n126 = call <instrlib>:"C63800 Set PF of AC RLC.vi"("error in (no error)"=w370, "PF of RLC"=w368, "Instrument Handle"=w367) -> ("error out"=w369:errorcluster)  [unwired: 7 in, 1 out]
              }
              frame "RLC (AC)" {
                w397 = T3 [enum."Current", enum."Current Peak", enum."Current Limit", enum."Capacitance", enum."Inductance", enum."Parallel Resistance", enum."Series Resistance"] items=["Power", "Power Limit", "Current", "Current Peak", "Current Limit", "Voltage", "AC Resistance", "DC Resistance", "Frequency", "Crest Factor", "Power Factor", "RLC Power Factor", "Rise Slew Rate", "Fall Slew Rate", "Capacitance", "Inductance", "Parallel Resistance", "Series Resistance"] ("RangeCheck")
                w403 = 4 items=["CC", "CP", "CV", "CR", "RLC", "RLCP", "INRUSH", "RECT"] ("Load Mode")
                n127 = call-dynamic "CheckSettings.vi"("ChromaAcLoad in"=w398, "RangeCheck"=w397, "error in (no error)"=w400) -> ("error out"=w386:errorcluster)  [unwired: 6 in, 1 out]
                n128 = call <instrlib>:"C63800 Set AC or DC Mode.vi"("error in (no error)"=w386, "Select AC_DC Mode"=FALSE, "Instrument Handle"=w383) -> ("error out"=w385:errorcluster, "Instrument Handle out"=w384:refnum<k15>)  [unwired: 7 in]
                n129 = call <instrlib>:"C63800 Set Load Mode.vi"("error in (no error)"=w385, "Load Mode"=w403, "Instrument Handle"=w384) -> ("error out"=w402:errorcluster, "Instrument Handle out"=w401:refnum<k15>)  [unwired: 7 in]
                n130 = Unbundle By Name(w406) -> ("Load Current (A/Arms)"=w393:dbl, "LC/RLC Mode.Capacitance (uF)"=w417:i32, "LC/RLC Mode.Inductance (uH)"=w414:i32, "LC/RLC Mode.Parallel Resistance (Ohm)"=w409:dbl, "LC/RLC Mode.Series Resistance (Ohm)"=w408:dbl, "Load Current Limit (A/Arms)"=w388:dbl, "Load Current Peak Limit (A)"=w407:dbl)
                n131 = call <instrlib>:"C63800 Set AC or DC Mode.vi"("error in (no error)"=w402, "Select AC_DC Mode"=FALSE, "Instrument Handle"=w401) -> ("error out"=w399:errorcluster, "Instrument Handle out"=w405:refnum<k15>)  [unwired: 7 in]
                n132 = call <instrlib>:"C63800 Set Ip(max) of AC.vi"("error in (no error)"=w399, "Current Peak Max"=w407, "Instrument Handle"=w405) -> ("error out"=w392:errorcluster, "Instrument Handle out"=w391:refnum<k15>)  [unwired: 7 in]
                n133 = call <instrlib>:"C63800 Set Maximum RMS Current.vi"("error in (no error)"=w392, "Set Max RMS Current"=w388, "Instrument Handle"=w391) -> ("error out"=w390:errorcluster, "Instrument Handle out"=w389:refnum<k15>)  [unwired: 7 in]
                n134 = call <instrlib>:"C63800 Set RS of AC RLC.vi"("error in (no error)"=w390, "RS of RLC"=w408, "Instrument Handle"=w389) -> ("error out"=w411:errorcluster, "Instrument Handle out"=w410:refnum<k15>)  [unwired: 7 in]
                n135 = call <instrlib>:"C63800 Set RL of AC RLC.vi"("error in (no error)"=w411, "RL of RLC"=w409, "Instrument Handle"=w410) -> ("error out"=w412:errorcluster, "Instrument Handle out"=w413:refnum<k15>)  [unwired: 7 in]
                n136 = call <instrlib>:"C63800 Set Ls of AC RLC.vi"("error in (no error)"=w412, "Ls of RLC"=w414, "Instrument Handle"=w413) -> ("error out"=w416:errorcluster, "Instrument Handle out"=w415:refnum<k15>)  [unwired: 7 in]
                n137 = call <instrlib>:"C63800 Set C of AC RLC.vi"("error in (no error)"=w416, "The Value C"=w417, "Instrument Handle"=w415) -> ("error out"=w396:errorcluster, "Instrument Handle out"=w395:refnum<k15>)  [unwired: 7 in]
                n138 = call <instrlib>:"C63800 Set RMS Current.vi"("error in (no error)"=w396, "Set RMS Current"=w393, "Instrument Handle"=w395) -> ("error out"=w394:errorcluster)  [unwired: 7 in, 1 out]
              }
            }
          }
        }
      }
    }
    frame Error {
    }
  }
  "error out" <- w6
  "ChromaAcLoad out" <- w5
